vi "Picture.vi"() -> ()   [LabVIEW 2021]
panel:
  in  "stop":bool
  in  "Keep Previous Locations":bool
  out "2D Picture":picture
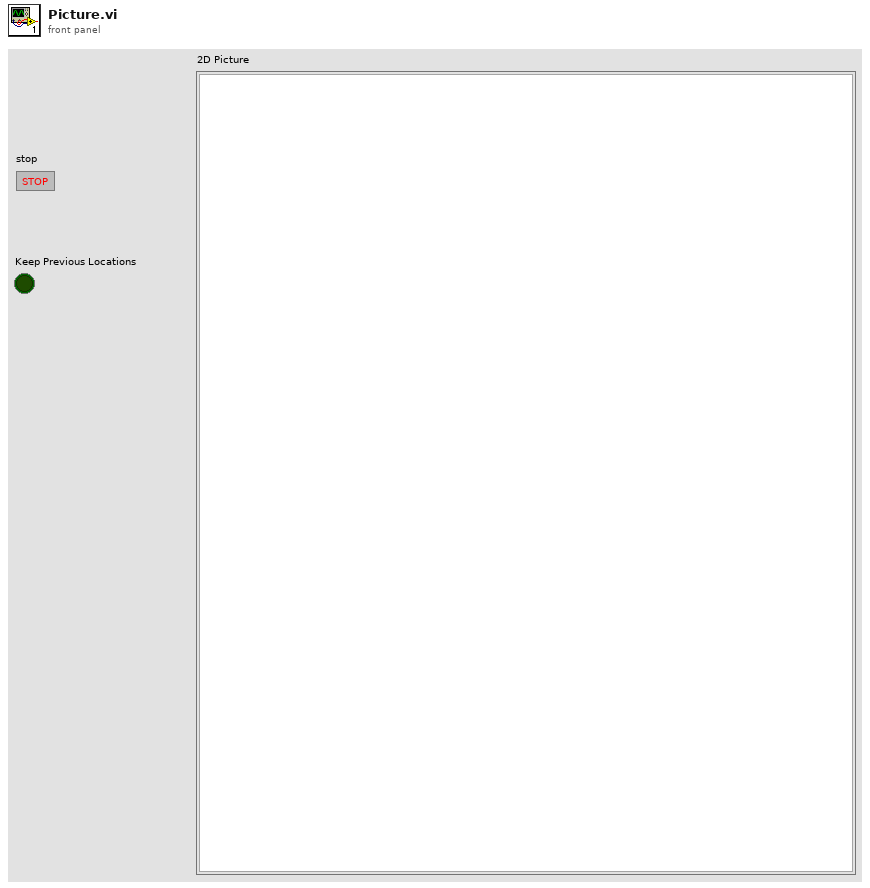
[diagram p1: front panel]
types:
  T1 = cluster{"Width":u16, "Style":enum32{"Solid", "Dash", "Dot", "DashDot", "DashDotDot"}}
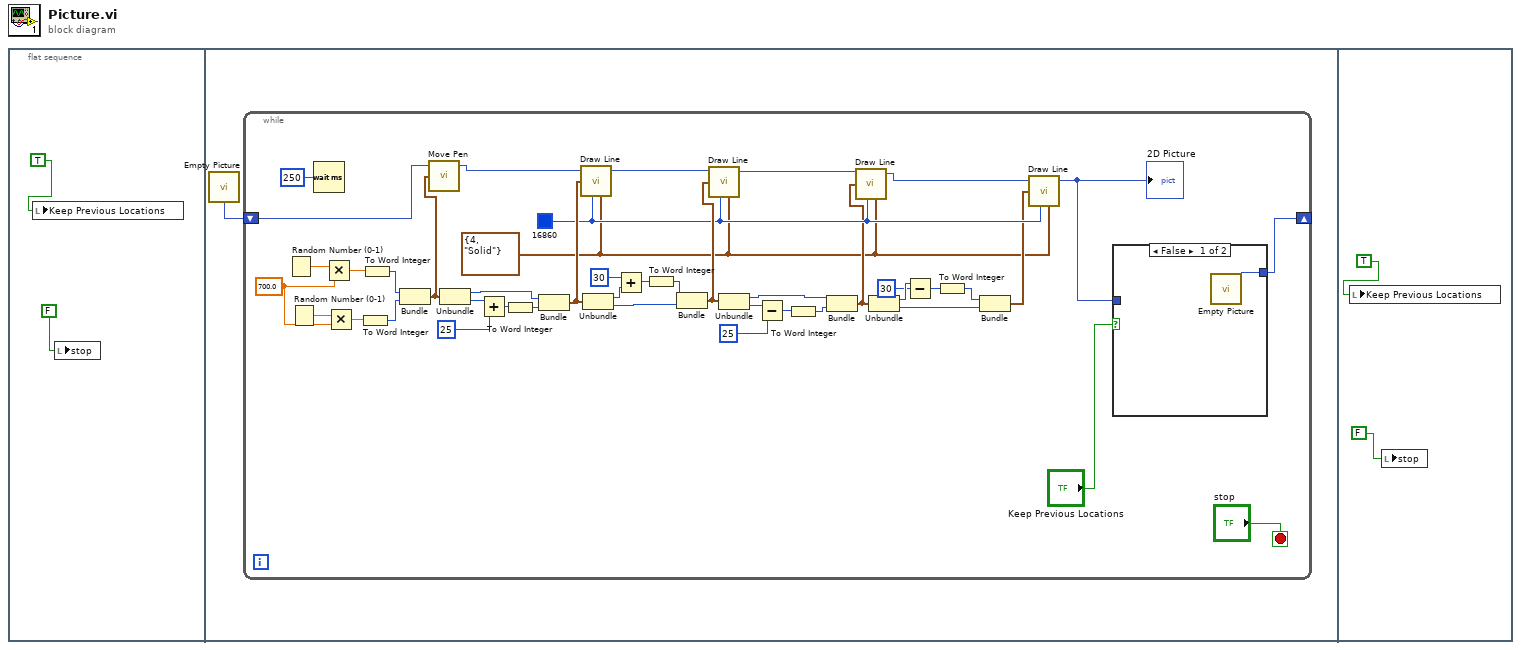
[diagram p0: block diagram]
diagram:
  n1 = flat-sequence {
    frame #0 {
      n2 = local write "Keep Previous Locations"(TRUE) -> ()
      n3 = local write "stop"(FALSE) -> ()
    }
    frame #1 {
      n4 = call "Empty Picture"() -> ("empty picture"=w3:picture)
      n5 = while {
        shift-right: [w4] -> _
        shift-left: w3 -> [w36]
        stop <- "stop" stop-if-true
        w5 = T1 {"Width"=4, "Style"=enum."Solid"} ("pen")
        w8 = u32 16860
        w43 = 700.0
        n6 = Random Number (0-1)() -> (number: 0 to 1=w45:dbl)
        n7 = Random Number (0-1)() -> (number: 0 to 1=w44:dbl)
        n8 = Wait (ms)(milliseconds to wait=u32 250) -> ()  [unwired: 1 out]
        n9 = Multiply(x=w45, y=w43) -> (x*y=w41:dbl)
        n10 = Multiply(x=w44, y=w43) -> (x*y=w40:dbl)
        n11 = To Word Integer(number=w40) -> (16bit integer=w38:i16)
        n12 = To Word Integer(number=w41) -> (16bit integer=w39:i16)
        n13 = Bundle(w39, w38) -> (w37:cluster{i16, i16})  [unwired: 1 in]
        n14 = call <vilib>:"Move Pen.vi"("new position"=w37, "picture"=w36) -> ("new picture"=w29:picture)  [unwired: 3 in]
        n15 = Unbundle(w37) -> (w31:i16, w35:i16)
        n16 = Add(x=w35, y=i16 25) -> (x+y=w33:i16)
        n17 = To Word Integer(number=w33) -> (16bit integer=w32:i16)
        n18 = Bundle(w31, w32) -> (w30:cluster{i16, i16})  [unwired: 1 in]
        n19 = call <vilib>:"Draw Line.vi"("picture"=w29, "end point"=w30, "color(black)"=w8, "pen"=w5) -> ("new picture"=w13:picture)  [unwired: 5 in]
        n20 = Unbundle(w30) -> (w28:i16, w26:i16)
        n21 = Add(x=i16 30, y=w28) -> (x+y=w25:i16)
        n22 = To Word Integer(number=w25) -> (16bit integer=w24:i16)
        n23 = Bundle(w24, w26) -> (w9:cluster{i16, i16})  [unwired: 1 in]
        n24 = call <vilib>:"Draw Line.vi"("picture"=w13, "end point"=w9, "color(black)"=w8, "pen"=w5) -> ("new picture"=w12:picture)  [unwired: 5 in]
        n25 = Unbundle(w9) -> (w19:i16, w23:i16)
        n26 = Subtract(x=w23, y=i16 25) -> (x-y=w21:i16)
        n27 = To Word Integer(number=w21) -> (16bit integer=w20:i16)
        n28 = Bundle(w19, w20) -> (w7:cluster{i16, i16})  [unwired: 1 in]
        n29 = call <vilib>:"Draw Line.vi"("picture"=w12, "end point"=w7, "color(black)"=w8, "pen"=w5) -> ("new picture"=w11:picture)  [unwired: 5 in]
        n30 = Unbundle(w7) -> (w18:i16, w14:i16)
        n31 = Subtract(x=w18, y=i16 30) -> (x-y=w16:i16)
        n32 = To Word Integer(number=w16) -> (16bit integer=w15:i16)
        n33 = Bundle(w15, w14) -> (w6:cluster{i16, i16})  [unwired: 1 in]
        n34 = call <vilib>:"Draw Line.vi"("picture"=w11, "end point"=w6, "color(black)"=w8, "pen"=w5) -> ("new picture"=w10:picture)  [unwired: 5 in]
        "2D Picture" <- w10
        n35 = case shown="False" "Keep Previous Locations" {
          tunnel: [w48 w49] -> w4
          tunnel: w10 -> [_ w49]
          frame False {
            n36 = call "Empty Picture"() -> ("empty picture"=w48:picture)
          }
          frame True {
          }
        }
      }
    }
    frame #2 {
      n37 = local write "Keep Previous Locations"(TRUE) -> ()
      n38 = local write "stop"(FALSE) -> ()
    }
  }
